vi "BRig_dataLC_Cue2_PreR_OnOff_l1.vi"() -> (2 "output_Cue2_PreR_OnOff":i32)   [LabVIEW 2014]
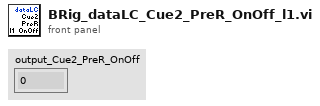
[diagram p1: front panel]
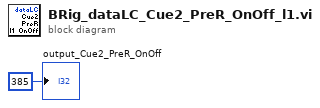
[diagram p0: block diagram]
diagram:
  "output_Cue2_PreR_OnOff" <- 385 ("output_iBlock")
